vi "step3 TestIfMiddleLayerSolved.vi"(8 "error in (no error)":errorcluster, 11 "cube in":T1) -> (0 "error out":errorcluster, 2 "middle layer solved?":bool)   [LabVIEW 2011]
uses:
  Typedef/cube.ctl
  Typedef/face.ctl
  Typedef/cube rotate direction.ctl
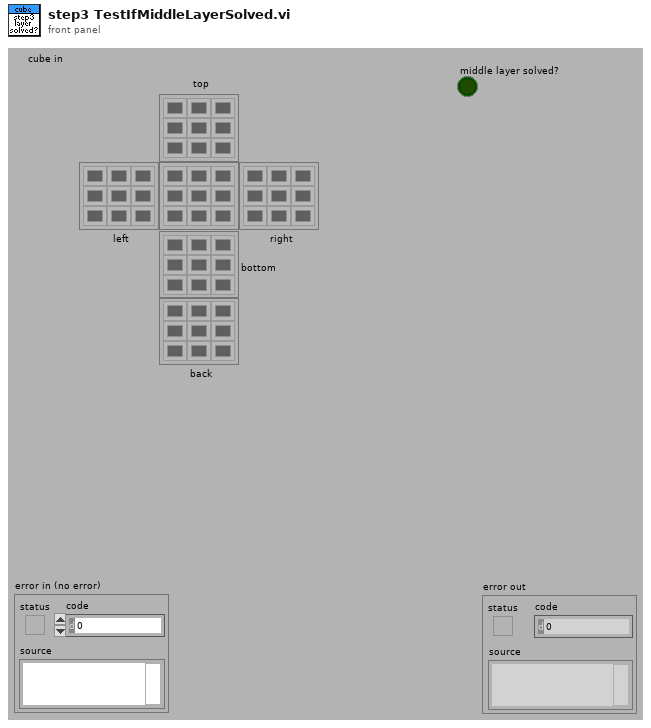
[diagram p1: front panel]
types:
  T1 = typedef "cube.ctl" = cluster{"top":T2, "left":T2, "right":T2, "bottom":T2, "back":T2, "front":T2}
  T2 = typedef "face.ctl" = u32[][]
  T3 = typedef "cube rotate direction.ctl" = enum16{"up", "down", "left", "right"}
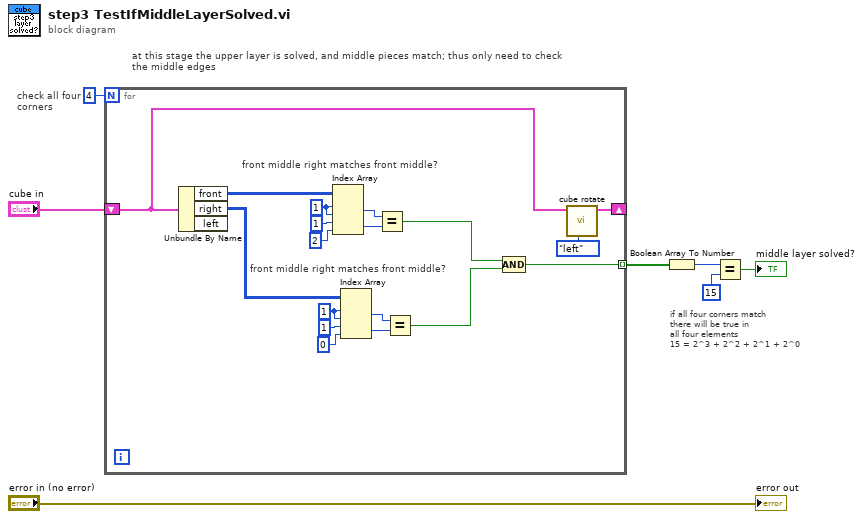
[diagram p0: block diagram]
diagram:
  # "check all four\ncorners"
  # "if all four corners match\nthere will be true in\nall four elements\n15 = 2^3 + 2^2 + 2^1 + 2^0"
  # "at this stage the upper layer is solved, and middle pieces match; thus only need to check\nthe middle edges"
  n1 = for {
    N: 4 -> [_]
    shift-right: [w20] -> _
    shift-left: "cube in" -> [w21]
    tunnel: [w22] -> w5 mode=indexing
    w11 = 1 ("index (row)")
    w24 = 1 ("index (row)")
    # "front middle right matches front middle?"
    # "front middle right matches front middle?"
    n2 = Unbundle By Name(w21) -> ("front"=w25:T2, "right"=w10:T2)  [unwired: 1 out]
    n3 = Index Array(array=w25, index (row) #1=w24, index (col) #1=w24, index (row) #2=1 ("index (row)"), index (col) #2=2 ("index (row)")) -> (element #1=w17:u32, element #2=w16:u32)
    n4 = Index Array(array=w10, index (row) #1=w11, index (col) #1=w11, index (row) #2=1 ("index (row)"), index (col) #2=0 ("index (row)")) -> (element #1=w14:u32, element #2=w15:u32)
    n5 = Equal?(x=w17, y=w16) -> (x = y?=w9:bool)
    n6 = Equal?(x=w14, y=w15) -> (x = y?=w8:bool)
    n7 = Compound Arithmetic op=AND(w9, w8) -> (w22:bool)
    n8 = call "cube rotate.vi"("cube rotation direction"=cube_rotate_direction."left", "cube in"=w21) -> ("cube out"=w20:T1)  [unwired: 8 in, 1 out]
  }
  n9 = Boolean Array To Number(Boolean array=w5) -> (number=w4:u32)
  n10 = Equal?(x=w4, y=u32 15) -> (x = y?=→"middle layer solved?":bool)
  "error out" <- "error in (no error)"
